vi "Helium3 Temperature 2 Pressure.vi"(11 "He3 Temperature (K)":dbl=0.4 format="%_6f") -> (3 "He3 Pressure (mbar)":dbl format="%#_5e")   [LabVIEW 2021]
uses:
  <vilib>/Analysis/polynomials.llb/Scalar Polynomial Evaluation (DBL).vi
  <vilib>/Analysis/NI_AALPro.lvlib
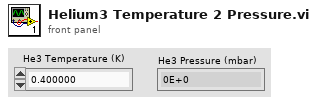
[diagram p1: front panel]
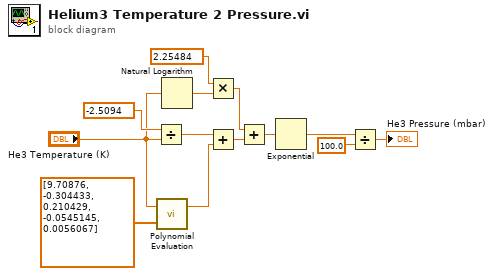
[diagram p0: block diagram]
diagram:
  n1 = Divide(x=-2.5094, y="He3 Temperature (K)") -> (x/y=w11:dbl)
  n2 = call-poly <vilib>:"Polynomial Evaluation.vi"("P(x)"=dbl[] [9.70876, -0.304433, 0.210429, -0.0545145, 0.0056067], "a"="He3 Temperature (K)") -> ("P(a)"=w10:dbl)  [unwired: 1 out]
  n3 = Natural Logarithm(1:"He3 Temperature (K)") -> (0:w8:dbl)
  n4 = Multiply(x=2.25484 ("y"), y=w8) -> (x*y=w6:dbl)
  n5 = Add(x=w11, y=w10) -> (x+y=w5:dbl)
  n6 = Add(x=w6, y=w5) -> (x+y=w4:dbl)
  n7 = Exponential(1:w4) -> (0:w3:dbl)
  n8 = Divide(x=w3, y=100.0) -> (x/y=→"He3 Pressure (mbar)":dbl)
